vi "PQfetchResultData.vi"(0 "conn":u32, 1 "res":u32, 5 "error in":errorcluster) -> (14 "conn_out":u32, 15 "res_out":u32, 16 "Data":string[][](array[string]), 17 "PQnTuples":u32, 18 "PQnFields":u32, 19 "error out":errorcluster)   [LabVIEW 2017, in "libpqutility.lvlib"]
doc: "Fetch Result Data from DatabaseRequest into String Array.\nSee PostgreSQL c-lib doku for further information."
uses:
  libpqutility.lvlib
  libpqlv/libpqlv.lvlib
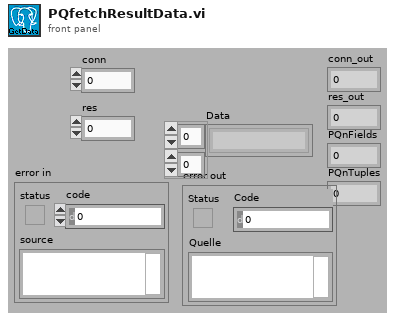
[diagram p1: front panel]
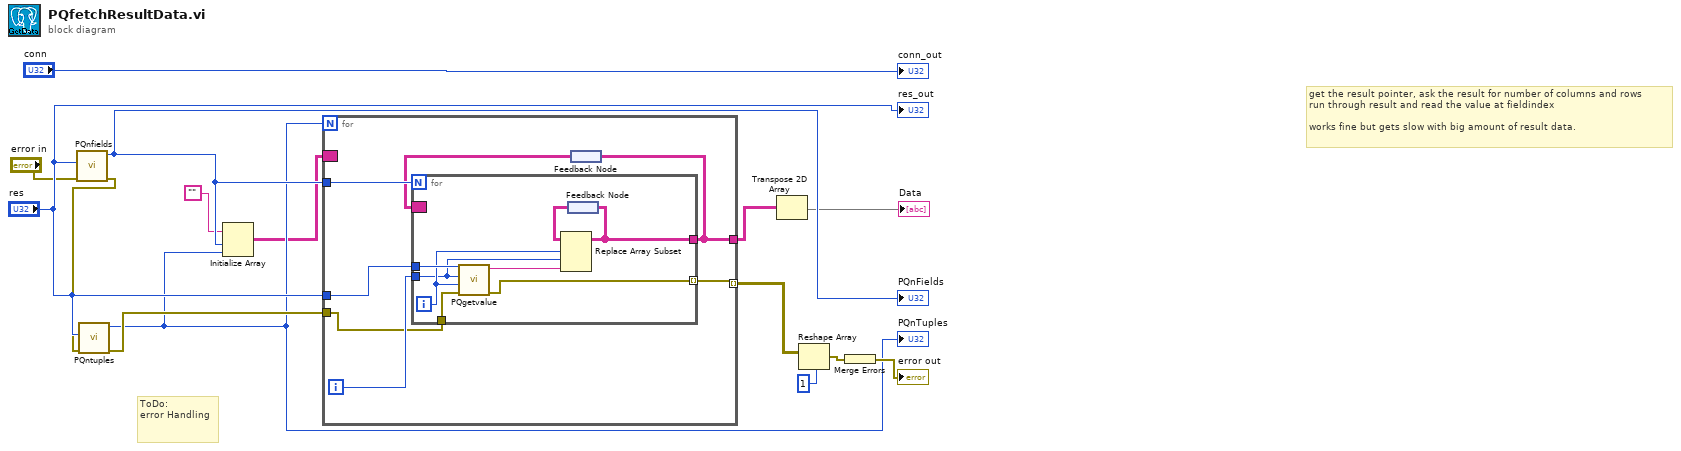
[diagram p0: block diagram]
diagram:
  # "ToDo:\nerror Handling"
  # "get the result pointer, ask the result for number of columns and rows\nrun through result and read the value at fieldindex\n\nworks fine but gets slow with big amount of result data."
  n1 = call "PQnfields.vi"("error in (no error)"="error in", "res"="res") -> ("error out"=w12:errorcluster, "PQnFields"=w6:u32)  [unwired: 8 in]
  "PQnFields" <- w6
  n2 = call "PQntuples.vi"("error in (no error)"=w12, "res"="res") -> ("error out"=w11:errorcluster, "PQnTuples"=w4:u32)  [unwired: 8 in]
  "PQnTuples" <- w4
  n3 = Initialize Array("", w6, w4) -> (w2:string[][])
  n4 = for {
    N: w4 -> [_]
    tunnel: "res" -> [w22]
    tunnel: w6 -> [w19]
    tunnel: w11 -> [w20]
    tunnel: [w18] -> w10 mode=indexing
    tunnel: [w17] -> w3
    border: w2 -> [_]
    i -> [w21]
    n5 = feedback #1() -> (w16:string[][])
    n6 = for {
      N: w19 -> [_]
      tunnel: w22 -> [w30]
      tunnel: w21 -> [w26]
      tunnel: w20 -> [w29]
      tunnel: [w28] -> w18 mode=indexing
      tunnel: [w24] -> w17
      border: w16 -> [_]
      i -> [w27]
      n7 = call "PQgetvalue.vi"("error in (no error)"=w29, "column_number"=w27, "row_number"=w26, "res"=w30) -> ("error out"=w28:errorcluster, "field_value"=w25:string)  [unwired: 6 in]
      n8 = feedback #2() -> (w23:string[][])
      n9 = Replace Array Subset(array=w23, new element=w25, index (row)=w27, index (col)=w26) -> (w24:string[][])
      n10 = feedback-in #2(w24) -> ()
    }
    n11 = feedback-in #1(w17) -> ()
  }
  n12 = Transpose 2D Array(2D array=w3) -> (transposed array=→"Data":string[][])
  n13 = Reshape Array(w10, 1 ("Dimensionsgröße")) -> (w8:errorcluster[])
  n14 = Merge Errors(w8) -> (→"error out":errorcluster)
  "res_out" <- "res"
  "conn_out" <- "conn"
